vi "GetDeviceConfig.vi"(8 "error in (no error)":errorcluster, 11 "Device":T1) -> (0 "error out":errorcluster, 1 "Sample Rate":dbl, 2 "Number of Dynamic Modules":i32, 3 "Name":string)   [LabVIEW 2017, in "McsaFpgaAcquisition.lvlib"]
uses:
  <vilib>/addons/InsightCM/Devices/Shared/Mcsa/McsaFpgaAcquisition/McsaFpgaAcquisition.lvlib
  <vilib>/addons/InsightCM/MessageBus/Base/controls/R2_Device.ctl
  <vilib>/addons/InsightCM/MessageBus/Base/controls/KeyValuePair.ctl
  <vilib>/addons/InsightCM/MessageBus/Base/controls/DeviceState.ctl
  <vilib>/addons/InsightCM/MessageBus/Base/controls/R2_DataGroup.ctl
  <vilib>/addons/InsightCM/MessageBus/Base/controls/OperatingState.ctl
  <vilib>/addons/InsightCM/MessageBus/Base/controls/Trigger.ctl
  <vilib>/addons/InsightCM/MessageBus/Base/controls/Condition.ctl
  <vilib>/addons/InsightCM/MessageBus/Base/controls/BurstModeTrigger.ctl
  <vilib>/addons/InsightCM/Utilities/PropertyHelpers/PropertyHelpers.lvlib
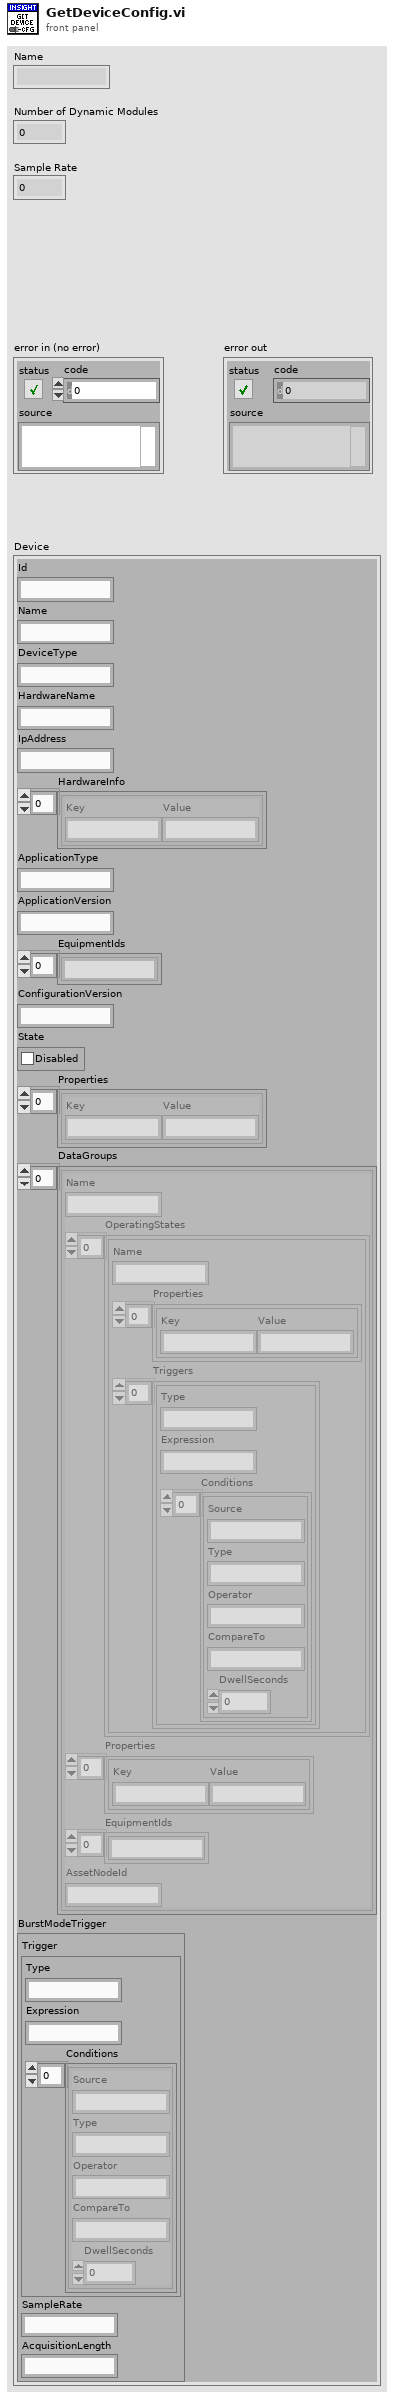
[diagram p1: front panel]
types:
  T1 = typedef "R2_Device.ctl" = cluster{"Id":string, "Name":string, "DeviceType":string, "HardwareName":string, "IpAddress":string, "HardwareInfo":T2[], "ApplicationType":string, "ApplicationVersion":string, "EquipmentIds":string[], "ConfigurationVersion":string, "State":T3, "Properties":T2[], "DataGroups":T4[], "BurstModeTrigger":T8}
  T2 = typedef "KeyValuePair.ctl" = cluster{"Key":string, "Value":string}
  T3 = typedef "DeviceState.ctl" = cluster{"Disabled":bool}
  T4 = typedef "R2_DataGroup.ctl" = cluster{"Name":string, "OperatingStates":T5[], "Properties":T2[], "EquipmentIds":string[], "AssetNodeId":string}
  T5 = typedef "OperatingState.ctl" = cluster{"Name":string, "Properties":T2[], "Triggers":T6[]}
  T6 = typedef "Trigger.ctl" = cluster{"Type":string, "Expression":string, "Conditions":T7[]}
  T7 = typedef "Condition.ctl" = cluster{"Source":string, "Type":string, "Operator":string, "CompareTo":string, "DwellSeconds":dbl}
  T8 = typedef "BurstModeTrigger.ctl" = cluster{"Trigger":T6, "SampleRate":string, "AcquisitionLength":string}
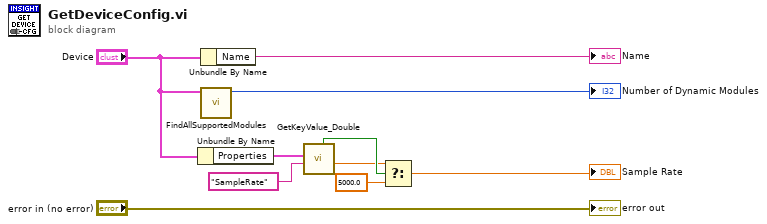
[diagram p0: block diagram]
diagram:
  n1 = Unbundle By Name("Device") -> ("Properties"=w3:T2[])
  n2 = Unbundle By Name("Device") -> ("Name"=→"Name":string)
  n3 = call <vilib>:"FindAllSupportedModules.vi"("Device Model"="Device") -> ("Number of Supported Modules"=→"Number of Dynamic Modules":i32)  [unwired: 9 in, 1 out]
  n4 = call <vilib>:"GetKeyValue_Double.vi"("key"="SampleRate", "key value pairs"=w3) -> ("value"=w1:dbl, "found"=w6:bool)  [unwired: 7 in, 1 out]
  n5 = Select(t=w1, s=w6, f=5000.0) -> (s? t:f=→"Sample Rate":dbl)
  "error out" <- "error in (no error)"
